vi "Choose Idle or Error State.vi"(5 "error in (no error)":errorcluster, 6 "Message Queue":refnum<queue>) -> ()   [LabVIEW 2020]
uses:
  Message Queue/test Message Queue.lvlib
  Message Queue/Enqueue Message (Single).vi
  Message Queue/Message Cluster.ctl
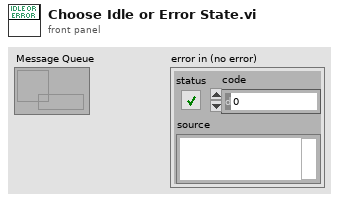
[diagram p1: front panel]
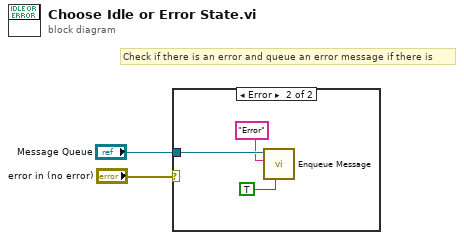
[diagram p0: block diagram]
diagram:
  # "Check if there is an error and queue an error message if there is"
  n1 = case shown="Error" "error in (no error)" {
    tunnel: "Message Queue" -> [_ w5]
    frame No Error {
    }
    frame Error {
      n2 = call-poly "Enqueue Message.vi"("Priority Message? (F)"=TRUE, "Message"="Error", "Message Queue"=w5) -> ()  [unwired: 7 in, 2 out]
    }
  }
